vi "Filter_Calcs.vi"(8 "FIFO Array in":refnum<queue>[][][](array[refnum]), 10 "Previous Detector Correlation":i32[][](array[numeric]), 11 "Current Detector output":i32[][](array[numeric])) -> (0 "FIFO Array out":refnum<queue>[][][](array[refnum]), 3 "Detector Correlation":i32[][](array[numeric]))   [LabVIEW 2015]
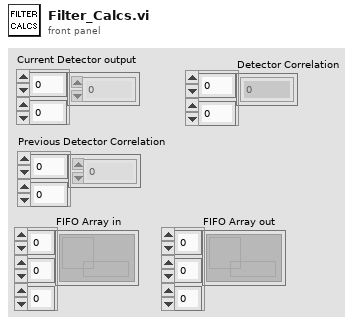
[diagram p1: front panel]
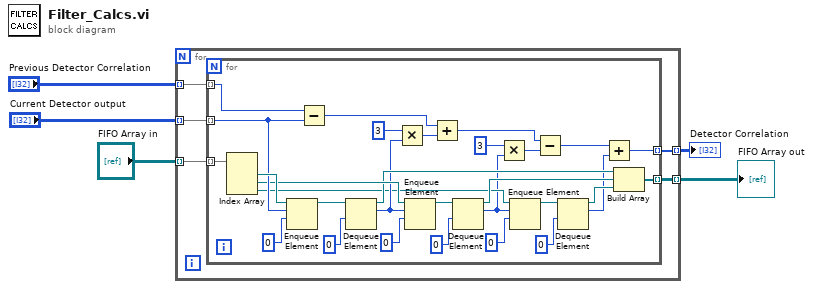
[diagram p0: block diagram]
diagram:
  n1 = for {
    tunnel: "FIFO Array in" -> [w8] mode=indexing
    tunnel: "Previous Detector Correlation" -> [w10] mode=indexing
    tunnel: "Current Detector output" -> [w9] mode=indexing
    tunnel: [w7] -> w2 mode=indexing
    tunnel: [w6] -> w1 mode=indexing
    n2 = for {
      tunnel: w10 -> [w37] mode=indexing
      tunnel: w9 -> [w36] mode=indexing
      tunnel: w8 -> [w40] mode=indexing
      tunnel: [w12] -> w7 mode=indexing
      tunnel: [w11] -> w6 mode=indexing
      n3 = Index Array(array=w40) -> (element #1=w39:refnum<queue>, element #2=w32:refnum<queue>, element #3=w20:refnum<queue>)  [unwired: 3 in]
      n4 = Enqueue Element(queue=w39, element=w36, timeout in ms (-1)=0) -> (queue out=w35:refnum<queue>)  [unwired: 1 in, 2 out]
      n5 = Subtract(x=w37, y=w36) -> (x-y=w28:i32)
      n6 = Dequeue Element(queue=w35, timeout in ms (-1)=0) -> (queue out=w31:refnum<queue>, element=w30:i32)  [unwired: 1 in, 2 out]
      n7 = Multiply(x=i16 3 ("n"), y=w30) -> (x*y=w27:i32)
      n8 = Enqueue Element(queue=w32, element=w30, timeout in ms (-1)=0) -> (queue out=w25:refnum<queue>)  [unwired: 1 in, 2 out]
      n9 = Add(x=w28, y=w27) -> (x+y=w16:i32)
      n10 = Dequeue Element(queue=w25, timeout in ms (-1)=0) -> (queue out=w21:refnum<queue>, element=w18:i32)  [unwired: 1 in, 2 out]
      n11 = Multiply(x=i16 3 ("n"), y=w18) -> (x*y=w17:i32)
      n12 = Enqueue Element(queue=w20, element=w18, timeout in ms (-1)=0) -> (queue out=w15:refnum<queue>)  [unwired: 1 in, 2 out]
      n13 = Subtract(x=w16, y=w17) -> (x-y=w14:i32)
      n14 = Dequeue Element(queue=w15, timeout in ms (-1)=0) -> (queue out=w22:refnum<queue>, element=w13:i32)  [unwired: 1 in, 2 out]
      n15 = Add(x=w14, y=w13) -> (x+y=w11:i32)
      n16 = Build Array(w31, w21, w22) -> (w12:refnum<queue>[])
    }
  }
  "Detector Correlation" <- w1
  "FIFO Array out" <- w2
